vi "Main.vi"() -> ()   [LabVIEW 2020]
uses:
  Libraries/Haptic IC Class/Haptic IC/Controls/IC I2C Clock Rate.ctl
  SubVIs/Serial/Controls/(Ctrl)Serial_FGV Function.ctl
  SubVIs/Mode Event/Controls/(Ctrl)Mode Event_FGV Function.ctl
  SubVIs/Control Data/Controls/(Ctrl)Control Data_Save or Load Control Data_Function.ctl
  Controls/(Ctrl)Launcher_RedNoah3 Edition.ctl
  <vilib>/Utility/miscctls.llb/LVPointTypeDef.ctl
  Libraries/Haptic IC Class/DW7800/DW7800.lvclass
  Libraries/Haptic IC Class/DW7802/DW7802.lvclass
  Libraries/Haptic IC Class/DW7912/DW7912.lvclass
  Libraries/Haptic IC Class/DW7914/DW7914.lvclass
  Libraries/Haptic IC Class/Haptic IC/Haptic IC.lvclass/Haptic IC.ctl
  Libraries/Haptic IC Class/Haptic IC/Accessors/Write ic type.vi
  Libraries/Haptic IC Class/Haptic IC/Accessors/Write i2c id.vi
  91ef870f-b17b-47a3-bf55-932f3be53e32.vi
  11f7903f-f19c-401a-86c5-9ea5b813f69c.vi
  Variables/(Var)RedNoah3 Info.vi
  <vilib>/Comparison/Equal/Equal Functor/Equal Functor.lvclass
  Libraries/Haptic IC Class/Haptic IC/Haptic IC.lvclass
  SubVIs/Serial/Instance VIs/(SubVI)Serial_Write-Read.vi
panel:
  in  "CP_I2c Clock Rate":T1=enum."1Mhz" caption="I2c Clock Rate"
  out "CP_Rednoah Pict":u8(ring)
  in  "CP_Vibration Scope":bool
  in  "CP_Retry":bool
  in  "CP_FW Update":bool
  in  "CP_I2C ID":u8(ring) caption="I2C ID :" items=["0x59 (0xB2)"=89]
  in  "CP_IC Type":u16(ring) caption="IC Type :" items=["DW7800", "Dw7802", "DW7912", "DW7914 (DW7917)"]
  in  "CP_Waveform Editor":bool
  out "CP_Rednoah Status":string caption="Status :"
  out "CP_Rednoah Ver":string caption="Ver. :"
  in  "CP_Rednoah Port":refnum<visa-resource-name> caption="Port :"
  in  "LP_Clear Log":bool
  out "LP_I2C Log":string caption="I2C Log"
  # "Haptic Studio"
  # "IC"
  # "Rednoah3"
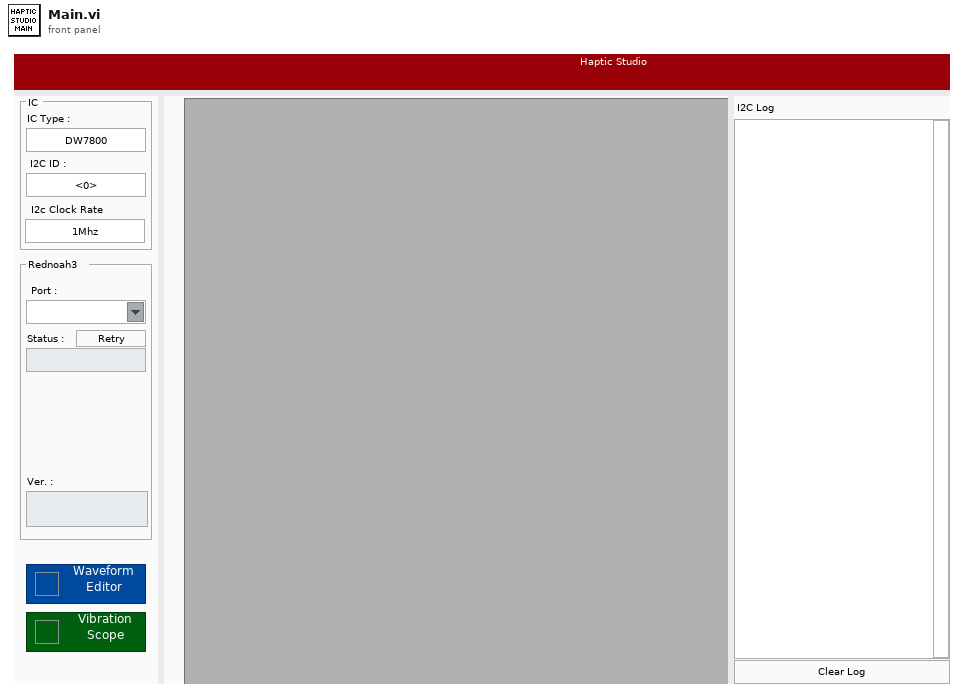
[diagram p1: front panel]
types:
  T1 = typedef "IC I2C Clock Rate.ctl" = enum8{"50khz", "100khz", "400khz", "1Mhz", "1.2Mhz"}
  T2 = typedef "(Ctrl)Control Data_Save or Load Control Data_Function.ctl" = enum16{"Save", "Load"}
  T3 = typedef "(Ctrl)Mode Event_FGV Function.ctl" = enum16{"Init", "Get Event Ref", "Gen Event", "Destroy"}
  T4 = typedef "(Ctrl)Serial_FGV Function.ctl" = enum16{"Initialize", "Read", "Read All", "Write", "Flush Buffer", "Get Ref.", "Close"}
  T5 = cluster{"Major":i32, "Minor":i32, "Patch":i32, "Build":i32}
  T6 = typedef "(Ctrl)Launcher_RedNoah3 Edition.ctl" = enum16{"Unknown", "Single Board", "Sensor Package"}
  T7 = typedef "LVPointTypeDef.ctl" = cluster{"Horizontal":i16, "Vertical":i16}
  T8 = enum8{"Enabled", "Disabled", "Disabled and Grayed Out"}
  T9 = typedef "LVRectTypeDef.ctl" = cluster{"Left":i16, "Top":i16, "Right":i16, "Bottom":i16}
  T10 = enum32{"Bad", "Idle", "Run top level", "Running"}
  T11 = typedef "LVStringsAndValuesArrayTypeDef_U8.ctl" = cluster{"String":string, "Value":u8}[]
  T12 = typedef "Haptic IC.lvclass/(Ctrl)IC Type.ctl" = enum8{"DW7800", "DW7802", "DW7912", "DW7914"}
  T13 = cluster{"BD SN":string, "BD FW Version":u32, "BD HW Version":enum8{"BBB 1.0", "BBB 1.1", "WBB 1.0", "reserved", "RedNoah3"}}
  T14 = enum32{"Invalid", "Standard", "Closed", "Hidden", "Minimized", "Maximized"}
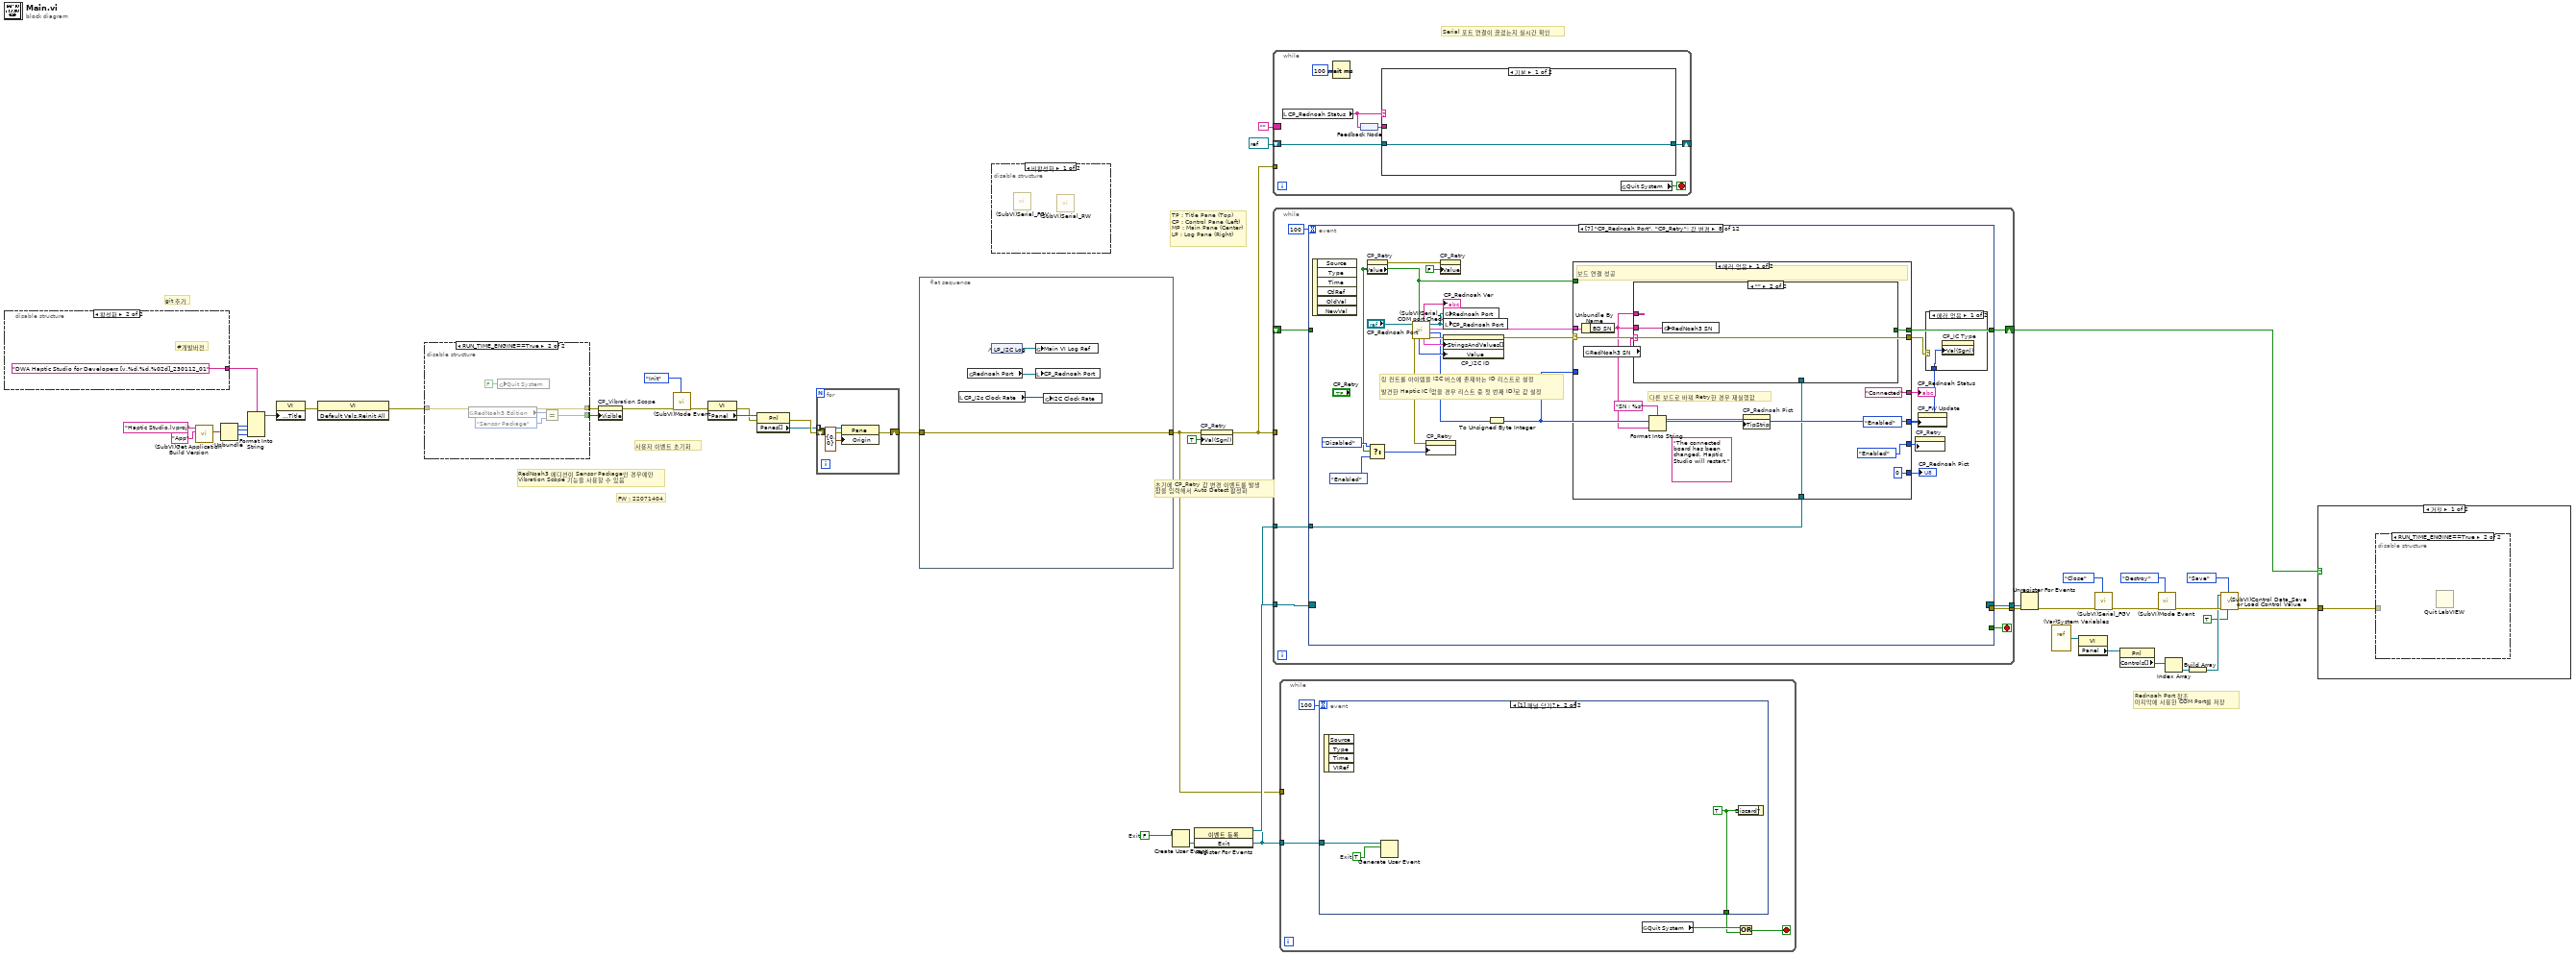
[diagram p0: block diagram]
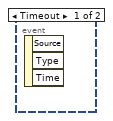
[diagram p3: hidden frame]
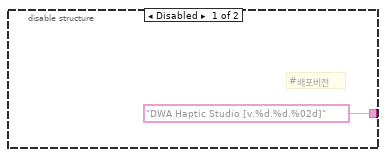
[diagram p4: hidden frame]
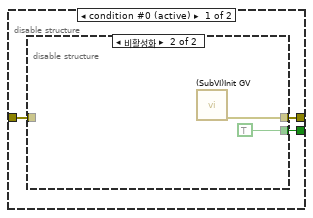
[diagram p5: hidden frame]
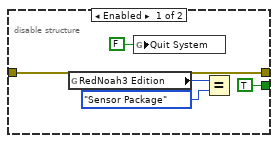
[diagram p6: hidden frame]
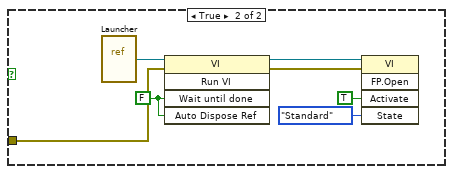
[diagram p8: hidden frame]
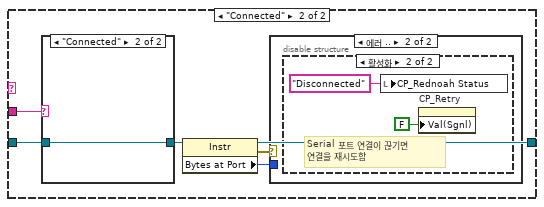
[diagram p9: hidden frame]
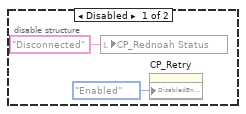
[diagram p11: hidden frame]
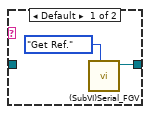
[diagram p12: hidden frame]
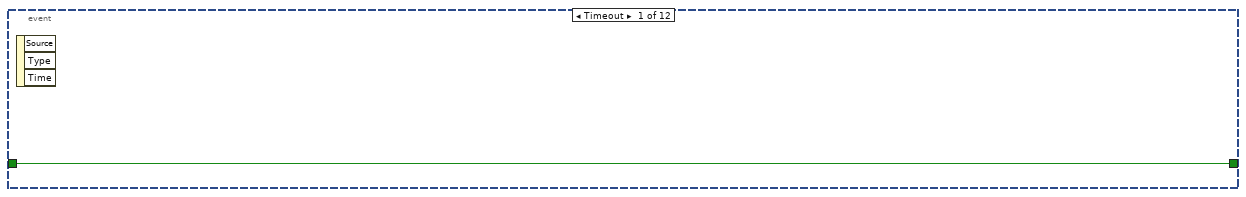
[diagram p13: hidden frame]
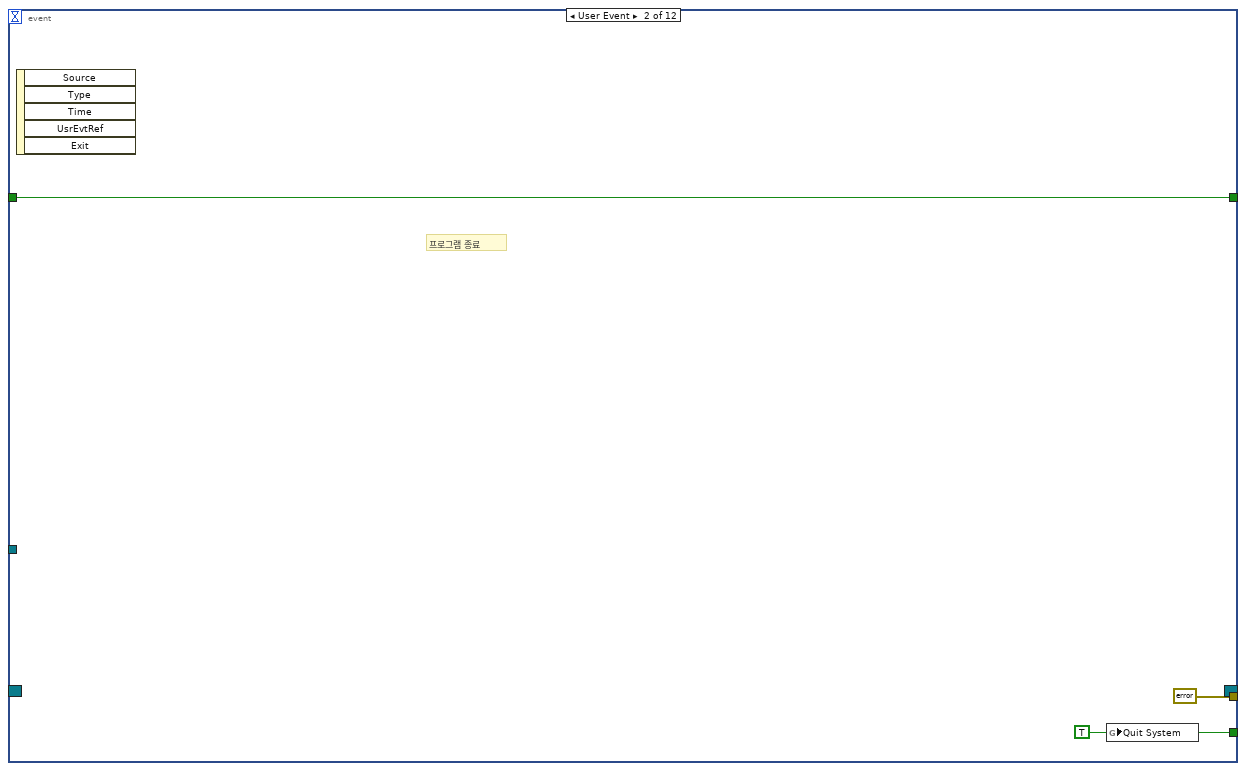
[diagram p14: hidden frame]
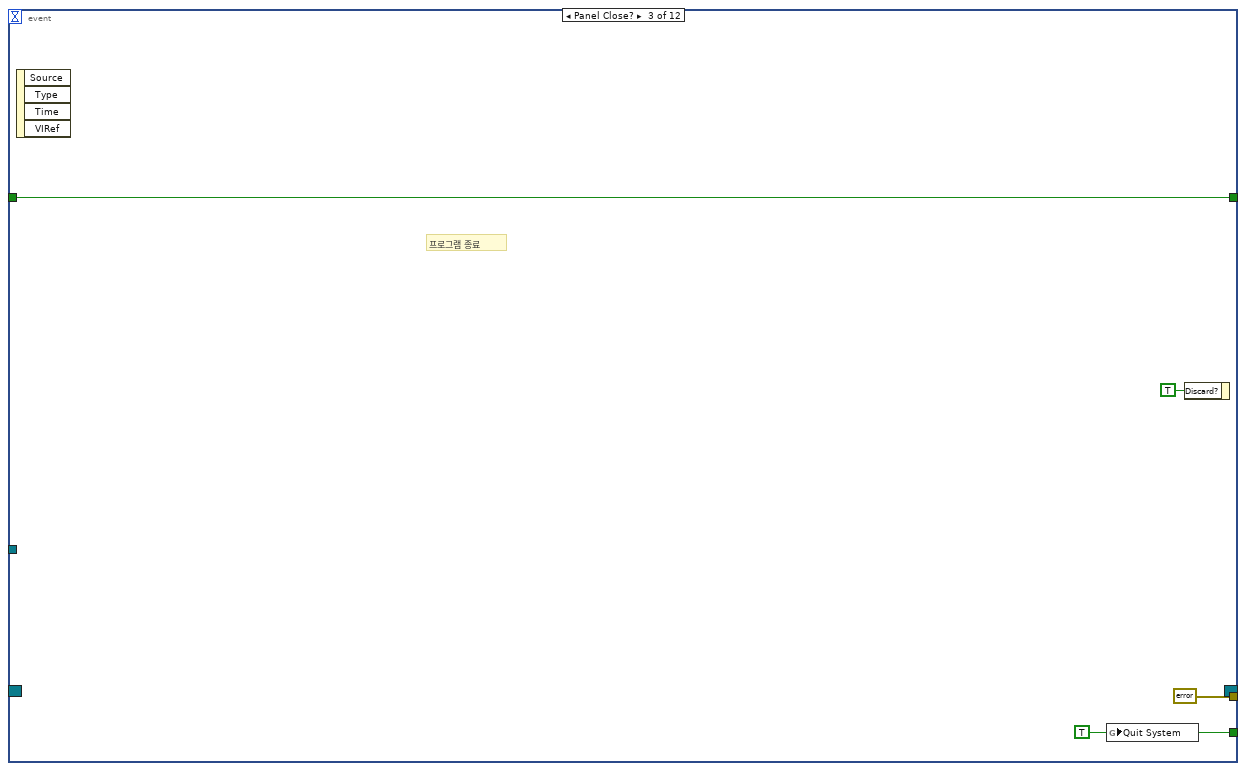
[diagram p15: hidden frame]
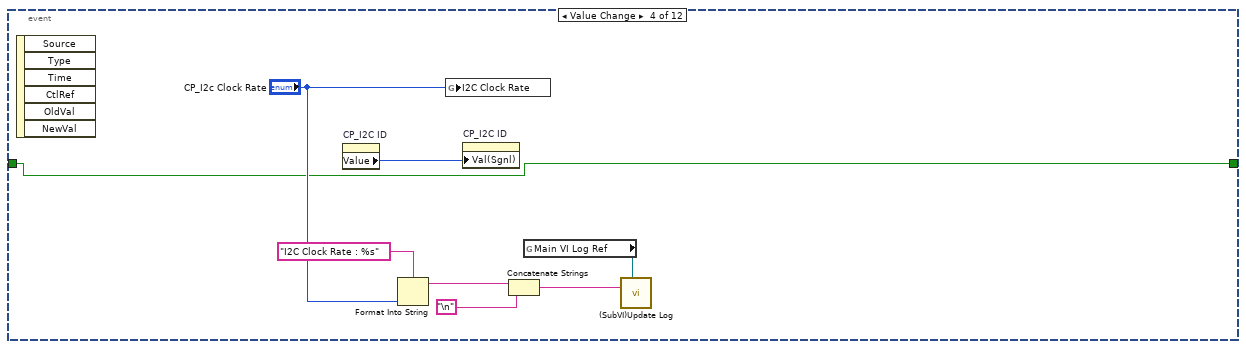
[diagram p16: hidden frame]
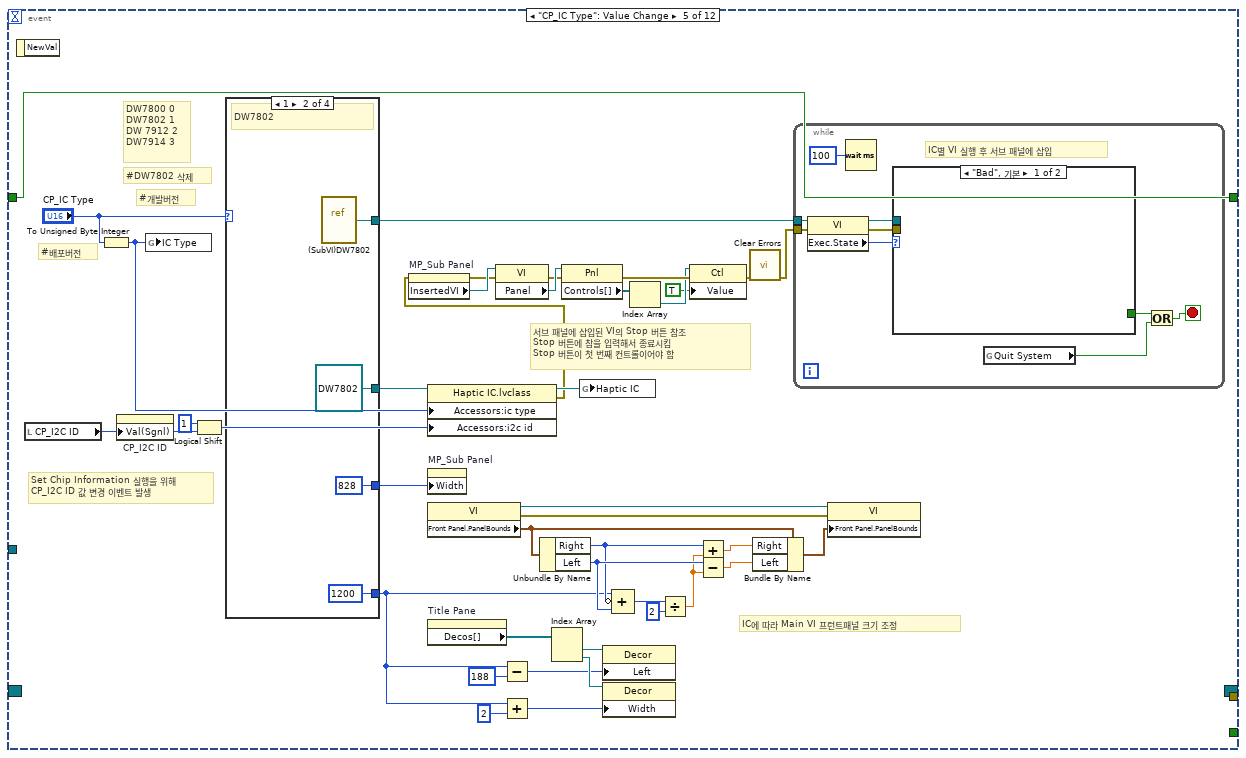
[diagram p17: hidden frame]
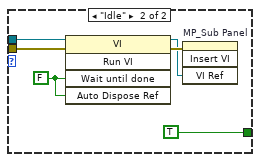
[diagram p18: hidden frame]
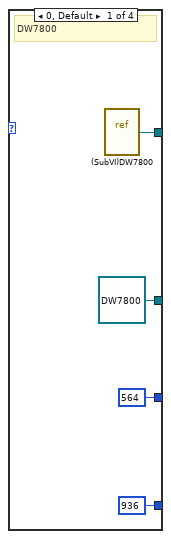
[diagram p19: hidden frame]
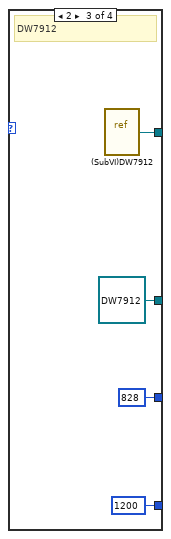
[diagram p20: hidden frame]
diagram:
  w6 = FALSE  # Exit
  # "git 추가"
  # "FW : 22071404"
  # "Rednoah Port 참조\n마지막에 사용한 COM Port를 저장"
  # "초기에 CP_Retry 값 변경 이벤트를 발생\n참을 입력해서 Auto Detect 활성화"
  # "Serial 포트 연결이 끊겼는지 실시간 확인"
  # "사용자 이벤트 초기화"
  # "RedNoah3 에디션이 Sensor Package인 경우에만\nVibration Scope 기능을 사용할 수 있음"
  # "TP : Title Pane (Top)\nCP : Control Pane (Left)\nMP : Main Pane (Center)\nLP : Log Pane (Right)"
  n1 = disable-structure shown="활성화" {
    disable-tunnel: ["DWA Haptic Studio [v.%d.%d.%02d]" ("포맷 문자열") "DWA Haptic Studio for Developers [v.%d.%d.%02d]_230112_01" ("포맷 문자열")] -> w12
    frame Disabled {
      # "#배포버전"
    }
    frame Enabled {
      # "#개발버전"
    }
  }
  n2 = call "(SubVI)Get Application Build Version.vi"("Build Specification Name"="App", "Project Filename"="Haptic Studio.lvproj") -> ("Version Numbers"=w16:T5)  [unwired: 7 in, 2 out]
  n3 = Unbundle(w16) -> ("Major"=w15:i32, "Minor"=w14:i32, "Patch"=w13:i32)  [unwired: 1 out]
  n4 = Format Into String(format string=w12, w15, w14, w13) -> (resulting string=w9:string)  [unwired: 2 in, 1 out]
  n5 = property class="VI"("Front Panel.Title"=w9) -> (error out=w8:errorcluster)  [unwired: 2 in, 1 out]
  n6 = invoke class="VI" method="Default Vals.Reinit All"(error in=w8) -> (error out=w18:errorcluster)  [unwired: 2 in, 2 out]
  n7 = disable-structure shown="RUN_TIME_ENGINE==True" {
    disable-tunnel: [w49 w60] -> w31
    disable-tunnel: [w48 w58] -> w28
    disable-tunnel: w18 -> [w47 w58]
    frame condition #0 (active) {
      n8 = disable-structure shown="비활성화" {
        disable-tunnel: [TRUE TRUE] -> w49
        disable-tunnel: [w52 w55] -> w48
        disable-tunnel: w47 -> [w52 _]
        frame Enabled {
          n9 = global read "(Var)RedNoah3 Info.vi" "RedNoah3 Edition"() -> (w53:T6)
          n10 = global write "(Var)System Variables.vi" "Quit System"(FALSE ("Quit System")) -> ()
          n11 = Equal?(x=w53, y=(Ctrl)Launcher_RedNoah3_Edition."Sensor Package") -> ()  [unwired: 1 out]
        }
        frame Disabled {
          n12 = call "(SubVI)Init GV.vi"() -> ("error out"=w55:errorcluster)  [unwired: 11 in]
        }
      }
    }
    frame condition #1 {
      n13 = global read "(Var)RedNoah3 Info.vi" "RedNoah3 Edition"() -> (w59:T6)
      n14 = global write "(Var)System Variables.vi" "Quit System"(FALSE ("Quit System")) -> ()
      n15 = Equal?(x=w59, y=(Ctrl)Launcher_RedNoah3_Edition."Sensor Package") -> (x = y?=w60:bool)
    }
  }
  n16 = property on="CP_Vibration Scope" class="Bool"(error in=w28, "Visible"=w31) -> (error out=w17:errorcluster)  [unwired: 1 in, 1 out]
  n17 = call "(SubVI)Mode Event.vi"("Function (Gen)"=(Ctrl)Mode_Event_FGV_Function."Init" ("Function"), "error in (no error)"=w17) -> ("error out"=w33:errorcluster)  [unwired: 8 in, 1 out]
  n18 = property class="VI"(error in=w33) -> (error out=w43:errorcluster, "Panel"=w44:refnum<vi>)  [unwired: 1 in, 1 out]
  n19 = property class="Pnl"(reference=w44, error in=w43) -> (error out=w42:errorcluster, "Panes[]"=w35:refnum<vi>[])  [unwired: 1 out]
  n20 = for {
    tunnel: w35 -> [w65] mode=indexing
    shift-right: [w62] -> w36
    shift-left: w42 -> [w63]
    n21 = property class="Pane"(reference=w65, error in=w63, "Origin"=T7 {"Horizontal"=0, "Vertical"=0} ("원점")) -> (error out=w62:errorcluster)  [unwired: 1 out]
  }
  n22 = flat-sequence {
    tunnel: [w69] -> w2
    tunnel: w36 -> [w69]
    frame #0 {
      n23 = local read "CP_I2c Clock Rate"() -> (w66:T1)
      n24 = global read "(Var)System Variables.vi" "Rednoah Port"() -> (w67:refnum<visa-resource-name>)
      n25 = control-ref of="LP_I2C Log"() -> (w68:refnum<vi>)
      n26 = global write "(Var)System Variables.vi" "Main VI Log Ref"(w68) -> ()
      n27 = local write "CP_Rednoah Port"(w67) -> ()
      n28 = global write "(Var)System Variables.vi" "I2C Clock Rate"(w66) -> ()
    }
  }
  n29 = disable-structure shown="비활성화" {
    frame Disabled {
      n30 = call "(SubVI)Serial_FGV.vi"() -> ()  [unwired: 9 in, 3 out]
      n31 = call-poly "(SubVI)Serial_RW.vi"() -> ()  [unwired: 9 in, 3 out]
    }
    frame Enabled {
    }
  }
  n32 = Create User Event(user event datatype=w6) -> (user event=w3:refnum<user-event>)  [unwired: 1 in, 1 out]
  n33 = register-events(w3) -> (reference out=w5:refnum<event-registration>)  [unwired: 2 in, 1 out]
  n34 = property on="CP_Retry" class="Bool (엄격한)"(error in=w2, "Val(Sgnl)"=TRUE ("값(신호)")) -> (error out=w7:errorcluster)  [unwired: 1 in, 1 out]
  n35 = while {
    tunnel: w7 -> [_]
    border: "" ("CP_Rednoah Status") -> [_]
    shift-right: [w73] -> _
    shift-left: refnum<visa-resource-name> refnum ("값(신호)") -> [w70]
    stop <- w72 stop-if-true
    n36 = local read "CP_Rednoah Status"() -> (w75:string)
    n37 = Wait (ms)(milliseconds to wait=u32 100 ("대기 시간 (ms)")) -> ()  [unwired: 1 out]
    n38 = feedback-in #1(w75) -> ()
    n39 = feedback #1() -> (w74:string)
    n40 = case shown="기본" w75 {
      tunnel: w74 -> [_ w81]
      tunnel: w70 -> [w76 w82]
      tunnel: [w76 w79] -> w73
      frame Default {
      }
      frame "Connected" {
        n41 = case shown="\"Connected\"" w81 {
          tunnel: w82 -> [_ w89]
          tunnel: [w87 w89] -> w80
          frame Default {
            n42 = call "(SubVI)Serial_FGV.vi"("Function"=(Ctrl)Serial_FGV_Function."Get Ref.") -> ("VISA resource name out"=w87:refnum<visa-resource-name>)  [unwired: 8 in, 2 out]
          }
          frame "Connected" {
          }
        }
        n43 = property class="Instr"(reference=w80) -> (reference out=w79:refnum<visa-resource-name>, error out=w78:errorcluster, "Bytes at Port"=w77:u32)  [unwired: 1 in]
        n44 = case shown="에러 .." w78 {
          tunnel: w77 -> [_ _]
          frame No Error {
          }
          frame Error {
            n45 = disable-structure shown="활성화" {
              frame Disabled {
                n46 = local write "CP_Rednoah Status"("Disconnected" ("CP_Rednoah Status")) -> ()
                n47 = property on="CP_Retry" class="Bool (엄격한)"("DisabledEnum"=T8."Enabled" ("비활성화")) -> ()  [unwired: 2 in, 2 out]
              }
              frame Enabled {
                # "Serial 포트 연결이 끊기면\n연결을 재시도함"
                n48 = local write "CP_Rednoah Status"("Disconnected" ("CP_Rednoah Status")) -> ()
                n49 = property on="CP_Retry" class="Bool (엄격한)"("Val(Sgnl)"=FALSE ("값(신호)")) -> ()  [unwired: 2 in, 2 out]
              }
            }
          }
        }
      }
    }
    n50 = global read "(Var)System Variables.vi" "Quit System"() -> (w72:bool)
  }
  n51 = while {
    tunnel: [w95] -> w41
    tunnel: w7 -> [_]
    tunnel: w5 -> [w93]
    tunnel: [w92] -> w4
    tunnel: w3 -> [w91]
    shift-right: [w94] -> w30
    shift-left: _ -> [w90]
    stop <- w96 stop-if-true
    n52 = event shown="[7] \"CP_Rednoah Port\", \"CP_Retry\": 값 변경" {
      selector: w93 -> [_ _ _ _ _ _ _ _ _ _ _ _]
      dyn-events: [_ _ _ _ _ _ _ _ _ _ _ _] -> w92
      timeout: 100 -> [_ _ _ _ _ _ _ _ _ _ _ _]
      tunnel: [_ w101 w105 _ _ _ _ _ _ _ _ _] -> w96
      tunnel: [_ errorcluster {"status"=FALSE, "code"=0, "source"=""} ("에러 상수") errorcluster {"status"=FALSE, "code"=0, "source"=""} ("에러 상수") _ _ _ _ _ _ _ _ _] -> w95
      tunnel: [w98 w99 w103 w106 w114 w186 w217 w251 w302 w314 w326 w345] -> w94
      tunnel: w91 -> [_ _ _ _ _ _ _ w249 _ _ _ _]
      tunnel: w90 -> [w98 w99 w103 w106 w114 w186 w217 _ w302 w314 w326 w345]
      event Timeout {
        n53 = event-data() -> ()  [unwired: 1 in, 3 out]
      }
      event User Event {
        w101 = TRUE
        # "프로그램 종료"
        n54 = event-data() -> ()  [unwired: 1 in, 5 out]
        n55 = global write "(Var)System Variables.vi" "Quit System"(w101) -> ()
      }
      event Panel Close? {
        w105 = TRUE
        # "프로그램 종료"
        n56 = event-data() -> ()  [unwired: 1 in, 4 out]
        n57 = global write "(Var)System Variables.vi" "Quit System"(w105) -> ()
        n58 = event-data("Discard?"=TRUE ("버림?")) -> ()  [unwired: 1 in, 1 out]
      }
      event Value Change {
        n59 = event-data() -> ()  [unwired: 1 in, 6 out]
        n60 = property on="CP_I2C ID" class="Ring (엄격한)"() -> ("Value"=w113:u8)  [unwired: 2 in, 2 out]
        n61 = Format Into String(format string="I2C Clock Rate : %s" ("포맷 문자열"), "CP_I2c Clock Rate") -> (resulting string=w109:string)  [unwired: 2 in, 1 out]
        n62 = global write "(Var)System Variables.vi" "I2C Clock Rate"("CP_I2c Clock Rate") -> ()
        n63 = property on="CP_I2C ID" class="Ring (엄격한)"("Val(Sgnl)"=w113) -> ()  [unwired: 2 in, 2 out]
        n64 = Concatenate Strings(w109, "\n") -> (w108:string)
        n65 = global read "(Var)System Variables.vi" "Main VI Log Ref"() -> (w112:refnum<vi>)
        n66 = call "(SubVI)Update Log.vi"("Log Ref"=w112, "Log"=w108) -> ()  [unwired: 8 in, 2 out]
      }
      event "CP_IC Type": Value Change {
        # "#배포버전"
        # "#개발버전"
        # "DW7800 0\nDW7802 1\nDW 7912 2\nDW7914 3"
        # "#DW7802 삭제"
        # "Set Chip Information 실행을 위해\nCP_I2C ID 값 변경 이벤트 발생"
        # "IC에 따라 Main VI 프런트패널 크기 조정"
        # "서브 패널에 삽입된 VI의 Stop 버튼 참조\nStop 버튼에 참을 입력해서 종료시킴\nStop 버튼이 첫 번째 컨트롤이어야 함"
        n67 = event-data() -> ()  [unwired: 1 in, 1 out]
        n68 = local read "CP_I2C ID"() -> (w120:u8)
        n69 = To Unsigned Byte Integer(number="CP_IC Type") -> (unsigned 8bit integer=w131:u8)
        n70 = property on="CP_I2C ID" class="Ring (엄격한)"("Val(Sgnl)"=w120) -> ()  [unwired: 2 in, 2 out]
        n71 = global write "(Var)System Variables.vi" "IC Type"(w131) -> ()
        n72 = Logical Shift(y=i16 1, x=w120) -> (x << y=w119:u8)
        n73 = case shown="1" "CP_IC Type" {
          tunnel: [w172 w176 w180 w184] -> w115
          tunnel: [refnum<class "DW7800.lvclass"> refnum ("DW7800.lvclass") refnum<class "DW7802.lvclass"> refnum ("DW7802.lvclass") refnum<class "DW7912.lvclass"> refnum ("DW7912.lvclass") refnum<class "DW7914.lvclass"> refnum ("DW7914.lvclass")] -> w153
          tunnel: [i16 936 i16 1200 i16 1200 i16 1200] -> w134
          tunnel: [u32 564 u32 828 u32 828 u32 828] -> w147
          frame 0, Default {
            # "DW7800"
            n74 = vi-ref "(SubVI)DW7800.vi"() -> (w172:refnum<vi>)
          }
          frame 1 {
            # "DW7802"
            n75 = vi-ref "(SubVI)DW7802.vi"() -> (w176:refnum<vi>)
          }
          frame 2 {
            # "DW7912"
            n76 = vi-ref "(SubVI)DW7912.vi"() -> (w180:refnum<vi>)
          }
          frame 3 {
            # "DW7914"
            n77 = vi-ref "(SubVI)DW7914.vi"() -> (w184:refnum<vi>)
          }
        }
        n78 = property class="Haptic IC.lvclass"(reference=w153, "Accessors:ic type"=w131, "Accessors:i2c id"=w119) -> (reference out=w152:refnum<class "Haptic IC.lvclass">, error out=w121:errorcluster)  [unwired: 1 in]
        n79 = property on="MP_Sub Panel" class="SubPnl"(error in=w121) -> (error out=w122:errorcluster, "InsertedVI"=w123:refnum<vi>)  [unwired: 1 in, 1 out]
        n80 = property on="MP_Sub Panel" class="SubPnl"("Width"=w147) -> ()  [unwired: 2 in, 2 out]
        n81 = property class="VI"() -> (reference out=w149:refnum<vi>, error out=w148:errorcluster, "Front Panel.PanelBounds"=w150:T9)  [unwired: 2 in]
        n82 = property on="Title Pane" class="Pane"() -> ("Decos[]"=w139:refnum<vi>[])  [unwired: 2 in, 2 out]
        n83 = property class="VI"(reference=w123, error in=w122) -> (error out=w124:errorcluster, "Panel"=w127:refnum<vi>)  [unwired: 1 out]
        n84 = Subtract(x=w134, y=i16 188) -> (x-y=w133:i16)
        n85 = Add(x=w134, y=i16 2) -> (x+y=w136:i16)
        n86 = Unbundle By Name(w150) -> ("Right"=w142:i16, "Left"=w144:i16)
        n87 = Index Array(array=w139) -> (element #1=w138:refnum<vi>, element #2=w137:refnum<vi>)  [unwired: 2 in]
        n88 = property class="Pnl"(reference=w127, error in=w124) -> (error out=w129:errorcluster, "Controls[]"=w126:refnum<vi>[])  [unwired: 1 out]
        n89 = global write "(Var)System Variables.vi" "Haptic IC"(w152) -> ()
        n90 = property class="Decor"(reference=w138, "Left"=w133) -> ()  [unwired: 1 in, 2 out]
        n91 = property class="Decor"(reference=w137, "Width"=w136) -> ()  [unwired: 1 in, 2 out]
        n92 = Compound Arithmetic op=ADD(w134, invert w142, w144) -> (w146:i16)
        n93 = Index Array(array=w126) -> (element=w128:refnum<vi>)  [unwired: 1 in]
        n94 = Divide(x=w146, y=i16 2) -> (x/y=w140:dbl)
        n95 = property class="Ctl"(reference=w128, error in=w129, "Value"=TRUE) -> (error out=w130:errorcluster)  [unwired: 1 out]
        n96 = Add(x=w142, y=w140) -> (x+y=w141:dbl)
        n97 = Subtract(x=w144, y=w140) -> (x-y=w143:dbl)
        n98 = call <vilib>:"Clear Errors.vi"("error in (no error)"=w130) -> ("error out"=w117:errorcluster)  [unwired: 5 in, 1 out]
        n99 = Bundle By Name(cluster=w150, "Right"=w141, "Left"=w143) -> (w116:T9)
        n100 = while {
          tunnel: w115 -> [w162]
          tunnel: w117 -> [w158]
          stop <- w155 stop-if-true
          # "IC별 VI 실행 후 서브 패널에 삽입"
          n101 = property class="VI"(reference=w162, error in=w158) -> (reference out=w161:refnum<vi>, error out=w160:errorcluster, "Exec.State"=w159:T10)
          n102 = Wait (ms)(milliseconds to wait=u32 100 ("대기 시간 (ms)")) -> ()  [unwired: 1 out]
          n103 = case shown="\"Bad\", 기본" w159 {
            tunnel: w161 -> [_ w167]
            tunnel: w160 -> [_ w166]
            tunnel: [_ TRUE] -> w157
            frame "Bad", Default {
            }
            frame "Idle" {
              w168 = FALSE ("완료될 때까지 기다림")
              n104 = invoke class="VI" method="Run VI"(reference=w167, error in=w166, "Wait until done"=w168, "Auto Dispose Ref"=w168) -> (reference out=w163:refnum<vi>, error out=w164:errorcluster)  [unwired: 1 in, 3 out]
              n105 = invoke on="MP_Sub Panel" class="SubPnl" method="Insert VI"(error in=w164, "VI Ref"=w163) -> ()  [unwired: 2 in, 4 out]
            }
          }
          n106 = global read "(Var)System Variables.vi" "Quit System"() -> (w154:bool)
          n107 = Or(x=w157, y=w154) -> (x .or. y?=w155:bool)
        }
        n108 = property class="VI"(reference=w149, error in=w148, "Front Panel.PanelBounds"=w116) -> ()  [unwired: 2 out]
      }
      event "CP_I2C ID": Value Change {
        # "RedNoah3에 Haptic IC의 I2C ID와 IC 타입 등을 전달"
        # "Haptic IC 데이터시트 문서에서 I2C ID를 7bit로 사용하기 때문에 UI에서 7bit로 보이게함\n\nRedNoah에서는 8bit(7bit + W)로 사용하기 때문에 코드에서는 1bit 시프트해서 사용"
        n109 = event-data() -> ()  [unwired: 1 in, 6 out]
        n110 = local read "CP_IC Type"() -> (w202:u16)
        n111 = global read "(Var)System Variables.vi" "Haptic IC"() -> (w205:refnum<class "Haptic IC.lvclass">)
        n112 = To Unsigned Byte Integer(number=w202) -> (unsigned 8bit integer=w201:u8)
        n113 = Logical Shift(y=i16 1, x="CP_I2C ID") -> (x << y=w193:u8)
        n114 = global write "(Var)System Variables.vi" "IC I2C ID"(w193) -> ()
        n115 = property class="Haptic IC.lvclass"(reference=w205, "Accessors:i2c id"=w193) -> (reference out=w204:refnum<class "Haptic IC.lvclass">)  [unwired: 1 in, 1 out]
        n116 = Logical Shift(y=i16 1, x="CP_I2C ID") -> (x << y=w191:u8)
        n117 = call "(SubVI)System Command_Set Chip Information.vi"("I2C ID"=w193, "Chip Type"=w201) -> ("error out"=w185:errorcluster)  [unwired: 8 in, 1 out]
        n118 = property on="CP_I2C ID" class="Ring (엄격한)"() -> ("StringsAndValues[]"=w188:T11)  [unwired: 2 in, 2 out]
        n119 = call <vilib>:"Clear Errors.vi"("error in (no error)"=w185) -> ()  [unwired: 5 in, 2 out]
        n120 = Format Into String(format string="0x%02x (0x%02x)" ("포맷 문자열"), "CP_I2C ID", w191) -> (resulting string=w198:string)  [unwired: 2 in, 1 out]
        n121 = Bundle(w198, "CP_I2C ID"="CP_I2C ID") -> (w189:cluster{string, "CP_I2C ID":u8})  [unwired: 1 in]
        n122 = global write "(Var)System Variables.vi" "Haptic IC"(w204) -> ()
        n123 = call "Search Unsorted 1D Array.vim"("element"=w189, "unsorted 1D array"=w188) -> ("index of element"=w197:i32)  [unwired: 9 in]
        n124 = Greater Or Equal To 0?(x=w197) -> (x >= 0?=w196:bool)
        n125 = case shown="참" w196 {
          tunnel: w188 -> [w208 w209]
          tunnel: w189 -> [w206 _]
          tunnel: [w207 w209] -> w195
          frame False {
            n126 = Insert Into Array(array=w208, new element=w206) -> (w207:T11)  [unwired: 1 in]
          }
          frame True {
          }
        }
        n127 = for {
          tunnel: [w214] -> w200 mode=indexing
          tunnel: w195 -> [w213] mode=indexing
          n128 = Unbundle By Name(w213) -> ("Value"=w211:u8)
          n129 = Logical Shift(y=i16 1, x=w211) -> (x << y=w210:u8)
          n130 = Format Into String(format string="0x%02x (0x%02x)" ("포맷 문자열"), w211, w210) -> (resulting string=w215:string)  [unwired: 2 in, 1 out]
          n131 = Bundle(w215, "Value"=w211) -> (w214:cluster{string, "Value":u8})  [unwired: 1 in]
        }
        n132 = property on="CP_I2C ID" class="Ring (엄격한)"("StringsAndValues[]"=w200) -> (error out=w194:errorcluster)  [unwired: 2 in, 1 out]
        n133 = property on="CP_I2C ID" class="Ring (엄격한)"(error in=w194, "Value"="CP_I2C ID") -> (error out=w187:errorcluster)  [unwired: 1 in, 1 out]
        n134 = call <vilib>:"Clear Errors.vi"("error in (no error)"=w187) -> ()  [unwired: 5 in, 2 out]
      }
      event "CP_I2C ID": Mouse Down? {
        # "CP_I2C ID 링 컨트롤을 클릭하는 순간 I2C ID를 스캔하여\n링 컨트롤 아이템을 업데이트함"
        n135 = event-data() -> ()  [unwired: 1 in, 1 out]
        n136 = property on="CP_I2C ID" class="Ring (엄격한)"() -> (error out=w228:errorcluster, "Value"=w220:u8)  [unwired: 2 in, 1 out]
        n137 = call "(SubVI)System Command_Find Auto I2C ID.vi"("error in (no error)"=w228) -> ("ID"=w229:u8[])  [unwired: 8 in, 2 out]
        n138 = for {
          tunnel: w229 -> [w234] mode=indexing
          tunnel: [w236] -> w219 mode=indexing
          n139 = Logical Shift(y=i16 -1, x=w234) -> (x << y=w235:u8)
          n140 = Format Into String(format string="0x%02x (0x%02x)" ("포맷 문자열"), w235, w234) -> (resulting string=w238:string)  [unwired: 2 in, 1 out]
          n141 = Bundle(w238, w235) -> (w236:cluster{string, u8})  [unwired: 1 in]
        }
        n142 = Logical Shift(y=i16 1, x=w220) -> (x << y=w224:u8)
        n143 = Format Into String(format string="0x%02x (0x%02x)" ("포맷 문자열"), w220, w224) -> (resulting string=w227:string)  [unwired: 2 in, 1 out]
        n144 = Bundle(w227, "Value"=w220) -> (w223:cluster{string, "Value":u8})  [unwired: 1 in]
        n145 = call "Search Unsorted 1D Array.vim"("element"=w223, "unsorted 1D array"=w219) -> ("index of element"=w226:i32)  [unwired: 9 in]
        n146 = Greater Or Equal To 0?(x=w226) -> (x >= 0?=w225:bool)
        n147 = case shown="참" w225 {
          tunnel: w219 -> [w232 w233]
          tunnel: w223 -> [w230 _]
          tunnel: [w231 w233] -> w218
          frame False {
            n148 = Insert Into Array(array=w232, new element=w230) -> (w231:cluster{string, u8}[])  [unwired: 1 in]
          }
          frame True {
          }
        }
        n149 = property on="CP_I2C ID" class="Ring (엄격한)"("StringsAndValues[]"=w218, "Value"=w220) -> ()  [unwired: 2 in, 2 out]
        n150 = event-data() -> ()  [unwired: 5 in, 1 out]
      }
      event "CP_Rednoah Port", "CP_Retry": Value Change {
        # "링 컨트롤 아이템을 I2C 버스에 존재하는 ID 리스트로 설정\n\n발견한 Haptic IC (없을 경우 리스트 중 첫 번째 ID)로 값 설정"
        n151 = event-data() -> ()  [unwired: 1 in, 6 out]
        n152 = property on="CP_Retry" class="Bool (엄격한)"() -> (error out=w255:errorcluster, "Value"=w242:bool)  [unwired: 2 in, 1 out]
        n153 = Select(t=T8."Disabled" ("비활성화"), s=w242, f=T8."Enabled" ("비활성화")) -> (s? t:f=w245:T8)
        n154 = property on="CP_Retry" class="Bool (엄격한)"("DisabledEnum"=w245) -> (error out=w246:errorcluster)  [unwired: 2 in, 1 out]
        n155 = call "(SubVI)Serial_COM port Check.vi"("Auto Detect?"=w242, "error in (no error)"=w246, "VISA resource name"="CP_Rednoah Port") -> ("error out"=w262:errorcluster, "IC Type"=w250:T12, "BD Version"=w241:T13, "VISA resource name out"=w253:refnum<visa-resource-name>, "I2C Slave ID"=w261:cluster{string, u8}[], "BD Info Str"=→"CP_Rednoah Ver":string, "Default I2C Slave ID"=w263:u8)  [unwired: 2 in]
        n156 = property on="CP_Retry" class="Bool (엄격한)"(error in=w255, "Value"=FALSE ("CP_Retry")) -> ()  [unwired: 1 in, 2 out]
        n157 = global write "(Var)System Variables.vi" "Rednoah Port"(w253) -> ()
        n158 = local write "CP_Rednoah Port"(w253) -> ()
        n159 = property on="CP_I2C ID" class="Ring (엄격한)"(error in=w262, "StringsAndValues[]"=w261, "Value"=w263) -> (error out=w252:errorcluster)  [unwired: 1 in, 1 out]
        n160 = To Unsigned Byte Integer(number=w250) -> (unsigned 8bit integer=w243:u8)
        n161 = case shown="에러 없음" w252 {
          selector: w252 -> [w269 w296]
          tunnel: ["Connected" ("f") "Disconnected" ("f")] -> w259
          tunnel: [T8."Enabled" ("f") T8."Disabled and Grayed Out" ("f")] -> w258
          tunnel: [T8."Enabled" ("f") T8."Enabled" ("f")] -> w257
          tunnel: w241 -> [w274 _]
          tunnel: [w272 _] -> w251
          tunnel: [u8 0 ("CP_Rednoah Pict") u8 1 ("CP_Rednoah Pict")] -> w254
          tunnel: w249 -> [w270 _]
          tunnel: [w269 w296] -> w244
          tunnel: w243 -> [_ w295]
          tunnel: w242 -> [_ _]
          frame No Error {
            (unwired) "The connected board has been changed. Haptic Studio will restart." ("메시지")
            # "다른 보드로 바꿔 Retry한 경우 재실행함"
            # "보드 연결 성공"
            n162 = Unbundle By Name(w274) -> ("BD SN"=w265:string)
            n163 = global read "(Var)RedNoah3 Info.vi" "RedNoah3 SN"() -> (w273:string)
            n164 = case shown="\"\"" w273 {
              selector: w273 -> [w283 _]
              tunnel: w265 -> [w284 w292]
              tunnel: [w282 _] -> w272
              tunnel: w265 -> [w281 _]
              tunnel: w270 -> [w277 _]
              frame Default {
                n165 = Empty String/Path?(string/path=w281) -> (empty?=w279:bool)
                n166 = Equal?(x=w284, y=w283) -> (x = y?=w280:bool)
                n167 = Or(x=w279, y=w280) -> (x .or. y?=w278:bool)
                n168 = case shown="참" w278 {
                  tunnel: [w286 _] -> w282
                  tunnel: w277 -> [w285 _]
                  frame False {
                    n169 = One Button Dialog(message="Board changed" ("메시지"), button name ("OK")="OK" ("버튼 이름(\"확인\")")) -> ()  [unwired: 1 out]
                    n170 = disable-structure shown="비활성화" {
                      disable-tunnel: [TRUE ("Quit System") _] -> w286
                      disable-tunnel: w285 -> [w289 _]
                      frame Disabled {
                        w290 = TRUE  # Exit
                        n171 = Generate User Event(user event=w289, event data cluster=w290) -> ()  [unwired: 2 in, 2 out]
                      }
                      frame Enabled {
                      }
                    }
                  }
                  frame True {
                  }
                }
              }
              frame "" {
                n172 = global write "(Var)RedNoah3 Info.vi" "RedNoah3 SN"(w292) -> ()
              }
            }
            n173 = Format Into String(format string="SN : %s" ("포맷 문자열"), w265) -> (resulting string=w267:string)  [unwired: 2 in, 1 out]
            n174 = property on="CP_Rednoah Pict" class="Ring (엄격한)"("TipStrip"=w267) -> ()  [unwired: 2 in, 2 out]
          }
          frame Error {
            # "보드 연결 실패"
            n175 = First Call?() -> (First Call?: T/F=w294:bool)
            n176 = case shown="참" w294 {
              tunnel: w295 -> [_ w301]
              frame False {
              }
              frame True {
                n177 = property on="CP_IC Type" class="Ring (엄격한)"("Val(Sgnl)"=w301) -> ()  [unwired: 2 in, 2 out]
              }
            }
            n178 = property on="CP_Rednoah Pict" class="Ring (엄격한)"("TipStrip"="" ("팁 상자")) -> ()  [unwired: 2 in, 2 out]
          }
        }
        "CP_Rednoah Status" <- w259
        "CP_Rednoah Pict" <- w254
        n179 = property on="CP_Retry" class="Bool (엄격한)"("DisabledEnum"=w257) -> ()  [unwired: 2 in, 2 out]
        n180 = property on="CP_FW Update" class="Bool"("DisabledEnum"=w258) -> ()  [unwired: 2 in, 2 out]
        n181 = case shown="에러 없음" w244 {
          tunnel: w243 -> [w264 _]
          frame No Error {
            n182 = property on="CP_IC Type" class="Ring (엄격한)"("Val(Sgnl)"=w264) -> ()  [unwired: 2 in, 2 out]
          }
          frame Error {
          }
        }
      }
      event "CP_Waveform Editor": Value Change {
        n183 = event-data() -> ()  [unwired: 1 in, 1 out]
        n184 = vi-ref "(SubVI)Waveform Editor.vi"() -> (w303:refnum<vi>)
        n185 = property class="VI"(reference=w303) -> (reference out=w306:refnum<vi>, error out=w305:errorcluster, "Exec.State"=w304:T10)  [unwired: 1 in]
        n186 = case shown="\"Idle\"" w304 {
          tunnel: [w307 w313] -> _
          tunnel: w306 -> [w307 w311]
          tunnel: w305 -> [w308 w310]
          tunnel: [w308 w309] -> _
          frame "Bad", Default {
          }
          frame "Idle" {
            w312 = FALSE ("완료될 때까지 기다림")
            n187 = invoke class="VI" method="Run VI"(reference=w311, error in=w310, "Wait until done"=w312, "Auto Dispose Ref"=w312) -> (reference out=w313:refnum<vi>, error out=w309:errorcluster)  [unwired: 1 in, 3 out]
          }
        }
      }
      event "CP_Vibration Scope": Value Change {
        n188 = event-data() -> ()  [unwired: 1 in, 6 out]
        n189 = vi-ref "(SubVI)Haptic Vibration Scope.vi"() -> (w315:refnum<vi>)
        n190 = property class="VI"(reference=w315) -> (reference out=w318:refnum<vi>, error out=w317:errorcluster, "Exec.State"=w316:T10)  [unwired: 1 in]
        n191 = case shown="\"Idle\"" w316 {
          tunnel: [w319 w325] -> _
          tunnel: w318 -> [w319 w323]
          tunnel: w317 -> [w320 w322]
          tunnel: [w320 w321] -> _
          frame "Bad", Default {
          }
          frame "Idle" {
            w324 = FALSE ("완료될 때까지 기다림")
            n192 = invoke class="VI" method="Run VI"(reference=w323, error in=w322, "Wait until done"=w324, "Auto Dispose Ref"=w324) -> (reference out=w325:refnum<vi>, error out=w321:errorcluster)  [unwired: 1 in, 3 out]
          }
        }
      }
      event "CP_FW Update": Value Change {
        # "업데이트 서버를 통해 FW를 자동으로 업데이트하게 되면서\n이 버튼은 사용하지 않음 (숨김처리)"
        n193 = event-data() -> ()  [unwired: 1 in, 6 out]
        n194 = call "파일 대화 상자"("prompt"="Select FW File...", "pattern (all files)"="*.bin", "pattern label"="bin") -> ("selected path"=w327:path, "cancelled"=w330:bool, "error out"=w329:errorcluster)  [unwired: 9 in, 1 out]
        n195 = Or(x=w330, y=w329) -> (x .or. y?=w328:bool)
        n196 = case shown="참" w328 {
          tunnel: w327 -> [w344 _]
          frame False {
            n197 = local read "CP_Rednoah Port"() -> (w343:refnum<visa-resource-name>)
            n198 = property class="Instr"(reference=w343, "Timeout"=u32 10000 ("General Settings:Timeout Value")) -> (reference out=w340:refnum<visa-resource-name>, error out=w341:errorcluster)  [unwired: 1 in]
            n199 = call "(SubVI)System Command_Firmware Update.vi"("popup"=TRUE, "error in (no error)"=w341, "FW File"=w344) -> ("error out"=w335:errorcluster)  [unwired: 7 in, 1 out]
            n200 = Select(t="Update Failed!!", s=w335, f="Update Complete") -> (s? t:f=w337:string)
            n201 = call <vilib>:"Clear Errors.vi"("error in (no error)"=w335) -> ("error out"=w336:errorcluster)  [unwired: 5 in, 1 out]
            n202 = One Button Dialog(message=w337) -> ()  [unwired: 1 in, 1 out]
            n203 = property on="CP_Rednoah Port" class="VISAName"(error in=w336, "Val(Sgnl)"=w340) -> ()  [unwired: 1 in, 2 out]
          }
          frame True {
          }
        }
      }
      event "LP_Clear Log": Value Change {
        n204 = event-data() -> ()  [unwired: 1 in, 6 out]
        "LP_I2C Log" <- ""
      }
    }
  }
  n205 = while {
    tunnel: w3 -> [w347]
    tunnel: w2 -> [_]
    stop <- w349 stop-if-true
    n206 = event shown="[1] 패널 닫기?" {
      selector: _ -> [_ _]
      dyn-events: _ -> [_ _]
      timeout: 100 -> [_ _]
      tunnel: [_ w354] -> w348
      tunnel: w347 -> [_ w353]
      event Timeout {
        n207 = event-data() -> ()  [unwired: 1 in, 3 out]
      }
      event Panel Close? {
        w352 = TRUE  # Exit
        w354 = TRUE ("버림?")
        n208 = event-data() -> ()  [unwired: 1 in, 4 out]
        n209 = Generate User Event(user event=w353, event data cluster=w352) -> ()  [unwired: 2 in, 2 out]
        n210 = event-data("Discard?"=w354) -> ()  [unwired: 1 in, 1 out]
      }
    }
    n211 = global read "(Var)System Variables.vi" "Quit System"() -> (w350:bool)
    n212 = Or(x=w350, y=w348) -> (x .or. y?=w349:bool)
  }
  n213 = Unregister For Events(event registration refnum=w4, error in=w41) -> (error out=w1:errorcluster)
  n214 = vi-ref "(Var)System Variables.vi"() -> (w26:refnum<vi>)
  n215 = property class="VI"(reference=w26) -> ("Panel"=w25:refnum<vi>)  [unwired: 1 in, 2 out]
  n216 = call "(SubVI)Serial_FGV.vi"("Function"=(Ctrl)Serial_FGV_Function."Close", "error in (no error)"=w1) -> ("error out"=w39:errorcluster)  [unwired: 7 in, 2 out]
  n217 = property class="Pnl"(reference=w25) -> ("Controls[]"=w24:refnum<vi>[])  [unwired: 1 in, 2 out]
  n218 = call "(SubVI)Mode Event.vi"("Function (Gen)"=(Ctrl)Mode_Event_FGV_Function."Destroy" ("Function"), "error in (no error)"=w39) -> ("error out"=w27:errorcluster)  [unwired: 8 in, 1 out]
  n219 = Index Array(array=w24) -> (element=w23:refnum<vi>)  [unwired: 1 in]
  n220 = Build Array(w23) -> (w22:refnum<vi>[])
  n221 = call "(SubVI)Control Data_Save or Load Control Value.vi"("Common? (f)"=TRUE, "Function"=(Ctrl)Control_Data_Save_or_Load_Control_Data_Function."Save", "error in (no error)"=w27, "Control Ref"=w22) -> ("error out"=w19:errorcluster)  [unwired: 7 in]
  n222 = case shown="거짓" w30 {
    tunnel: w19 -> [w355 w356]
    frame False {
      n223 = disable-structure shown="RUN_TIME_ENGINE==True" {
        disable-tunnel: w355 -> [_ _]
        frame condition #0 (active) {
        }
        frame condition #1 {
          n224 = Quit LabVIEW() -> ()  [unwired: 1 in]
        }
      }
    }
    frame True {
      w361 = FALSE ("완료될 때까지 기다림")
      n225 = vi-ref "Launcher.vi"() -> (w362:refnum<vi>)
      n226 = invoke class="VI" method="Run VI"(reference=w362, error in=w356, "Wait until done"=w361, "Auto Dispose Ref"=w361) -> (reference out=w360:refnum<vi>, error out=w359:errorcluster)  [unwired: 1 in, 3 out]
      n227 = invoke class="VI" method="FP.Open"(reference=w360, error in=w359, "Activate"=TRUE ("활성화?"), "State"=T14."Standard" ("상태")) -> ()  [unwired: 1 in, 5 out]
    }
  }
